vi "Logger.PGSQL.GetPublicEvents.vi"(8 "error in (no error)":errorcluster, 11 "Logger":refnum<class "Logger.PGSQL.lvclass">) -> (0 "error out":errorcluster, 2 "Public Events":T1, 3 "Logger out":refnum<class "Logger.PGSQL.lvclass">)   [LabVIEW 2019, in "Logger.PGSQL.lvlib" / "Logger.PGSQL.lvclass"]
doc: "---------------------------------------------------------------\nJKI State Machine Objects™\nhttp://jki.net/state-machine-objects/\nCopyright (C) 2005-2015, JKI <info@jki.net>\nALL RIGHTS RESERVEDJKI State Machine Objects (SMO) 1.0.0.4\nJKI - JKI\nCopyright (c) 2015, JKI"
uses:
  Logger.PGSQL.lvclass
  Typedefs/PublicEvents--Cluster.ctl
  Typedefs/PublicEvents--Logger.PGSQL.Read Variable.ctl
  Logger.PGSQL.lvclass/Logger.PGSQL.ctl
panel:
  # "For instructions on how to use the JKI State Machine Objects, examples and video tutorials, visit:\nhttp://jki.net/state-machine-objects/\n\nJKI State Machine Objects™\nhttp://jki.net/state-machine-objects/\nCopyright (C) 2005-2015, JKI <info@jki.net>\nALL RIGHTS RESERVED"
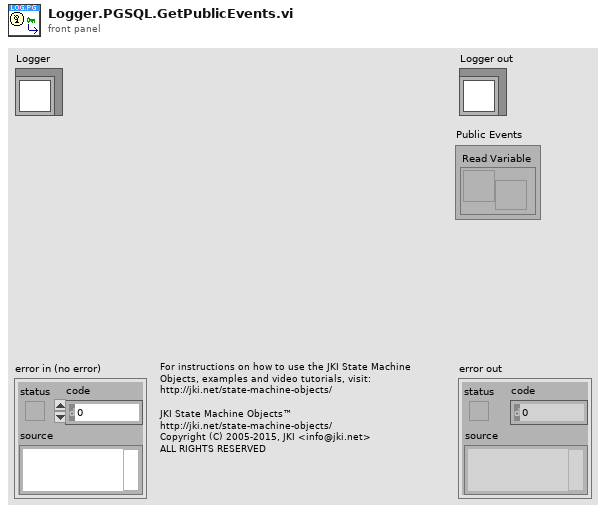
[diagram p1: front panel]
types:
  T1 = typedef "Logger.PGSQL.lvlib/Logger.PGSQL.lvclass/PublicEvents--Cluster.ctl" = cluster{"Read Variable":refnum<user-event>}
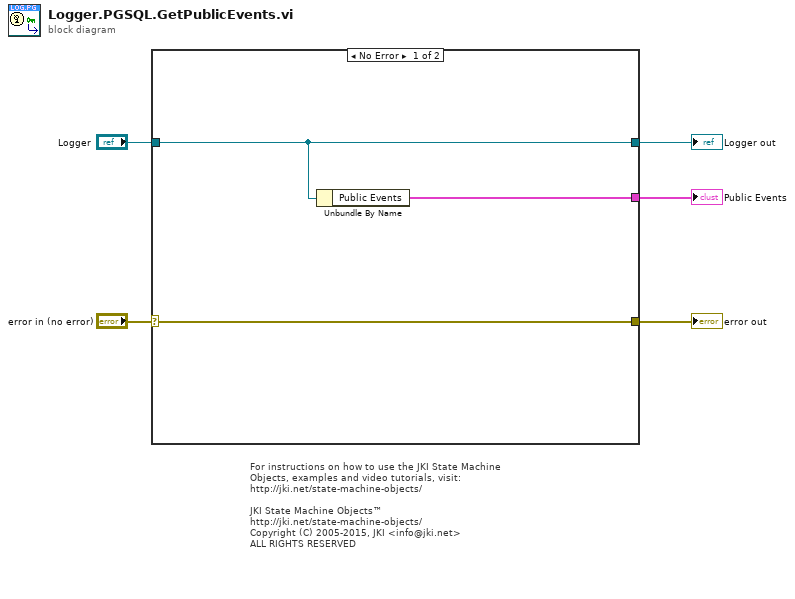
[diagram p0: block diagram]
diagram:
  # "For instructions on how to use the JKI State Machine Objects, examples and video tutorials, visit:\nhttp://jki.net/state-machine-objects/\n\nJKI State Machine Objects™\nhttp://jki.net/state-machine-objects/\nCopyright (C) 2005-2015, JKI <info@jki.net>\nALL RIGHTS RESERVED"
  n1 = case shown="No Error" "error in (no error)" {
    selector: "error in (no error)" -> [w7 w9]
    tunnel: "Logger" -> [w6 w10]
    tunnel: [w7 w9] -> w4
    tunnel: [w6 w10] -> w3
    tunnel: [w8 _] -> w1
    frame No Error {
      n2 = Unbundle By Name(w6) -> ("Public Events"=w8:T1)
    }
    frame Error {
    }
  }
  "error out" <- w4
  "Logger out" <- w3
  "Public Events" <- w1
